vi "Update Display UI.vi"(8 "error in (no error)":errorcluster, 11 "Display Console in":refnum<class "Display Console.lvclass">) -> (0 "error out":errorcluster, 3 "Display Console out":refnum<class "Display Console.lvclass">)   [LabVIEW 2019]
uses:
  Display Console.lvclass
  C:/Workspace/CLA/Elevator AF/Abstract Display Console Actor/Abstract Display Console Actor/Abstract Display Console.lvclass
  C:/Program Files (x86)/National Instruments/LabVIEW 2019/vi.lib/ActorFramework/Actor/Actor.lvclass
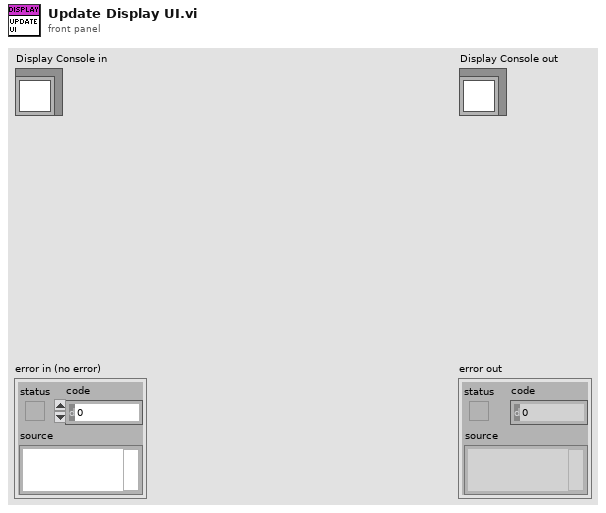
[diagram p1: front panel]
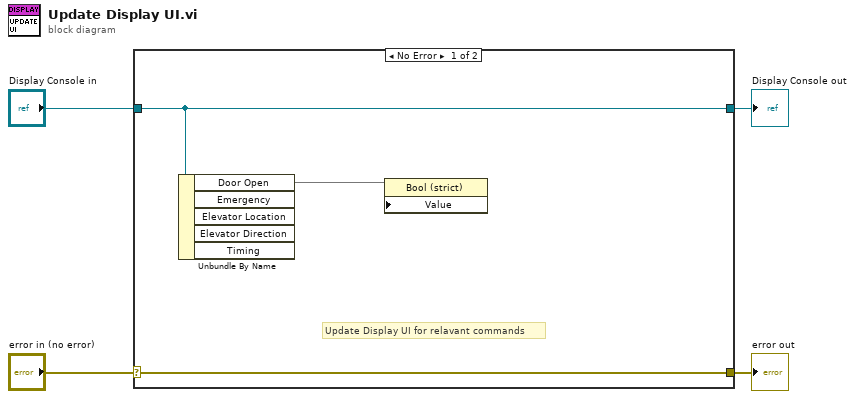
[diagram p0: block diagram]
diagram:
  n1 = case shown="No Error" "error in (no error)" {
    selector: "error in (no error)" -> [w7 w9]
    tunnel: [w7 w9] -> w3
    tunnel: [w6 w8] -> w1
    tunnel: "Display Console in" -> [w6 w8]
    frame No Error {
      # "Update Display UI for relavant commands"
      n2 = Unbundle By Name(w6) -> ("Door Open"=w5)  [unwired: 4 out]
      n3 = property class="Bool (strict)" props=["Value"](reference=w5) -> ()  [unwired: 2 in, 2 out]
    }
    frame Error {
    }
  }
  "error out" <- w3
  "Display Console out" <- w1
